vi "PTv3.0.vi"(8 "error in":errorcluster) -> ()   [LabVIEW 2017]
doc: "This VI runs in parallel to other tasks. It can contain as many user-defined periodic loops as you need. These can carry out PID or other sorts of timed response."
uses:
  <vilib>/Analysis/baseanly.llb/Mean (DBL).vi
  <vilib>/Rock Robotics/WPI/Utilities/WPI_GetSetVariantRefNum.vi
  <vilib>/Rock Robotics/Network Tables/NT Read Boolean.vi
  Robot Global Data.vi
  <vilib>/Rock Robotics/Network Tables/NT Write Number.vi
  <vilib>/Rock Robotics/Network Tables/NT Write Numeric Array.vi
  <vilib>/Analysis/NI_AALBase.lvlib
panel:
  out "Arrayval":dbl
  out "Accelerations":T1
  out "Joy Y":dbl(graph)
  out "Avg Y":dbl
  out "Mean":dbl(graph)
  out "Current Joy Y Value":dbl
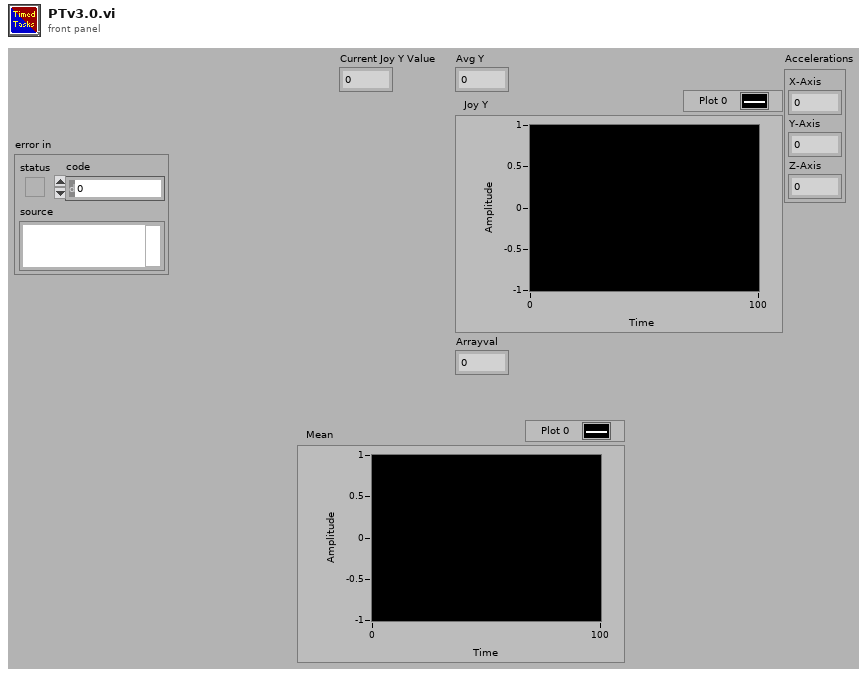
[diagram p1: front panel]
types:
  T1 = cluster{"X-Axis":dbl, "Y-Axis":dbl, "Z-Axis":dbl}
  T2 = typedef "WPI_JoystickDevRef.ctl" = cluster{"Device":T3}
  T3 = typedef "WPI_JoystickDeviceEnum.ctl" = enum16{"USB 0", "USB 1", "USB 2", "USB 3", "USB 4", "USB 5"}
  T4 = typedef "WPI_RobotDriveDevRef.ctl" = cluster{"DevStatus":errorcluster, "Motors[]":T5[], "Square Inputs":bool, "Max Output":dbl}
  T5 = typedef "WPI_MotorControlDeviceRef.ctl" = cluster{"DeviceStatus":errorcluster, "Type":T6, "PWM":cluster{"PWM Channel":T7, "DeadBand":T8}, "CAN":cluster{"Device Number":u8, "SetOutput VI Ref":variant, "GetOutput VI Ref":variant, "Enable VI Ref":variant, "Disable VI Ref":variant, "Data":variant}, "Invert":bool, "DIO PWM":cluster{"PWM \"Enable\" Channel":T7, "DIOChannel":T9, "PWM Rate":dbl}}
  T6 = typedef "WPI_MotorControlType.ctl" = enum16{"PWM", "CAN", "DIO PWM"}
  T7 = typedef "FPGA_DIOPWMChannel.ctl" = enum8{"PWM 0", "PWM 1", "PWM 2", "PWM 3", "PWM 4", "PWM 5", "PWM 6", "PWM 7", "PWM 8", "PWM 9", "PWM MXP 0", "PWM MXP 1", "PWM MXP 2", "PWM MXP 3", "PWM MXP 4", "PWM MXP 5", "PWM MXP 6", "PWM MXP 7", "PWM MXP 8", "PWM MXP 9", "Invalid"}
  T8 = typedef "WPI_PWMDeadband.ctl" = cluster{"Name":string, "maxPositivePwm":i32, "minPositivePwm":i32, "centerPwm":i32, "maxNegativePwm":i32, "minNegativePwm":i32, "angularRange":u16}
  T9 = typedef "FPGA_DIOChannel.ctl" = enum8{"DIO 0", "DIO 1", "DIO 2", "DIO 3", "DIO 4", "DIO 5", "DIO 6", "DIO 7", "DIO 8", "DIO 9", "DIO MXP 0", "DIO MXP 1", "DIO MXP 2", "DIO MXP 3", "DIO MXP 4", "DIO MXP 5", "DIO MXP 6", "DIO MXP 7", "DIO MXP 8", "DIO MXP 9", "DIO MXP 10", "DIO MXP 11", "DIO MXP 12", "DIO MXP 13", "DIO MXP 14", "DIO MXP 15", "SPI Port CS1", "SPI Port CS2", "SPI Port CS3", "SPI Port MISO", "SPI Port MOSI", "Invalid"}
  T10 = typedef "WPI_AccelerometerDevRef.ctl" = cluster{"DevStatus":errorcluster, "Scaling":T11, "Analog Channels":T12, "I2C Bus":T14, "SPI Bus":T15, "Accel Range":T16, "ADXL Axes":T17, "Handle":i32, "Device Address":u8, "Accel Type":enum16{"Analog", "ADXL345 I2C", "ADXL345 SPI", "Internal", "ADXL362 SPI"}}
  T11 = typedef "WPI_AccelerometerScaling.ctl" = cluster{"Gain (VoltsPerG)":dbl, "Center Voltage":dbl}
  T12 = typedef "WPI_AccelerometerAnalogChannels.ctl" = cluster{"X-Axis":T13, "Y-Axis":T13, "Z-Axis":T13}
  T13 = typedef "FPGA_AIChannel.ctl" = enum8{"AI 0", "AI 1", "AI 2", "AI 3", "AI MXP 0", "AI MXP 1", "AI MXP 2", "AI MXP 3", "Invalid"}
  T14 = typedef "i2c_bus.ctl" = enum16{"I2C On-Board", "I2C MXP", "Invalid"}
  T15 = typedef "spi_bus.ctl" = enum16{"SPI On-Board, CS0", "SPI On-Board, CS1", "SPI On-Board, CS2", "SPI On-Board, CS3", "SPI MXP", "Invalid"}
  T16 = typedef "ADXL345 Range.ctl" = u8
  T17 = typedef "WPI_AccelerometerADXL345 Axes.ctl" = cluster{"X-Axis":bool, "Y-Axis":bool, "Z-Axis":bool}
  T18 = typedef "WPI_GyroDevRef.ctl" = cluster{"DevStatus":errorcluster, "Analog Channel":T13, "Gain (VoltsPerDegree/Second)":dbl, "Gyro Type":enum16{"Analog", "XRS450"}, "Handle":i32, "SPI Bus":T15, "Device Found":bool, "Sample Rate":dbl, "Calibrate On Open":bool, "Offset":dbl}
  T19 = cluster{"JoystickDevRef":T2, "RobotDriveDevRef":T4}
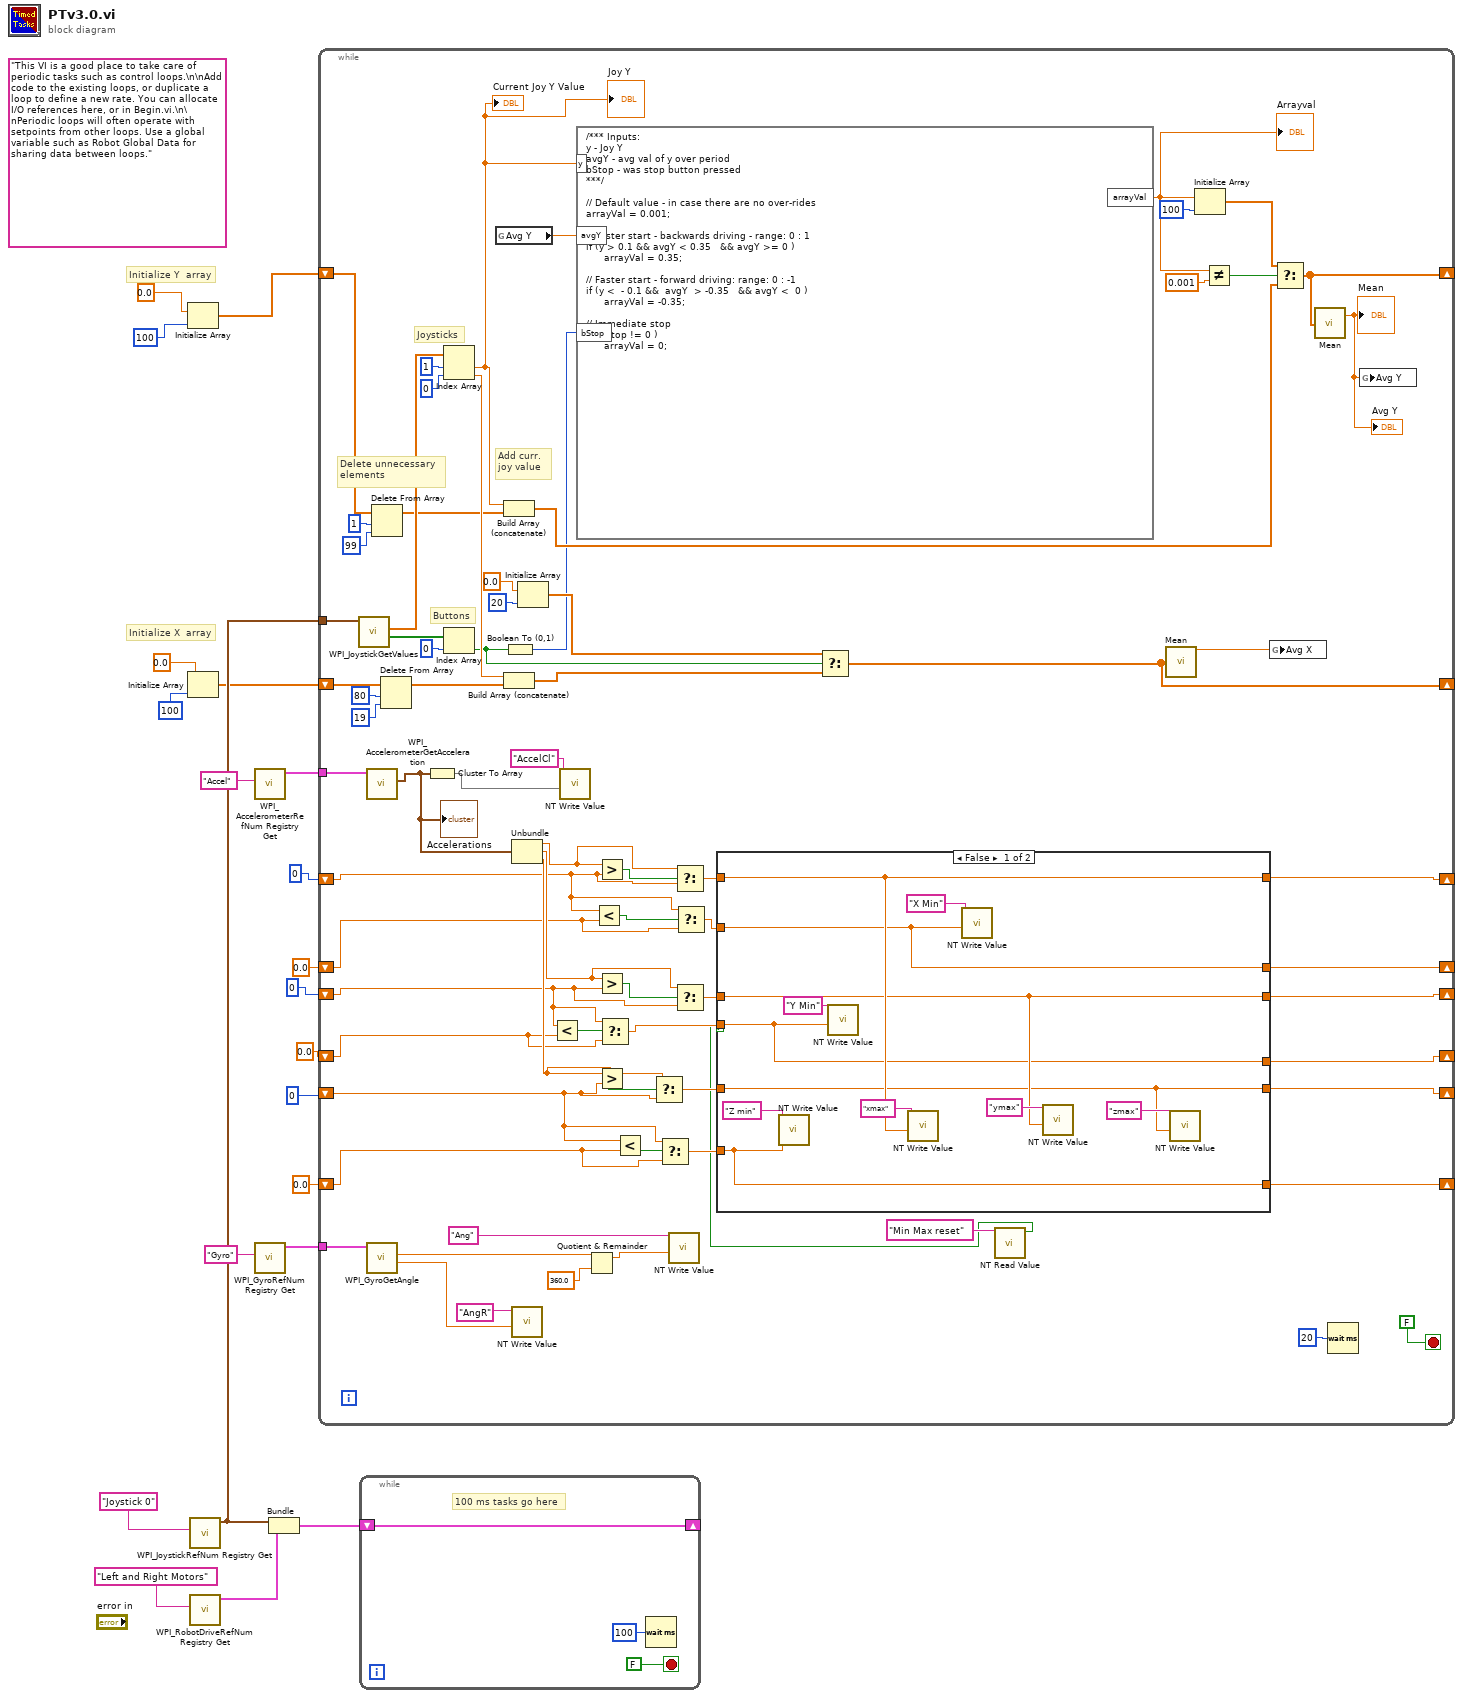
[diagram p0: block diagram]
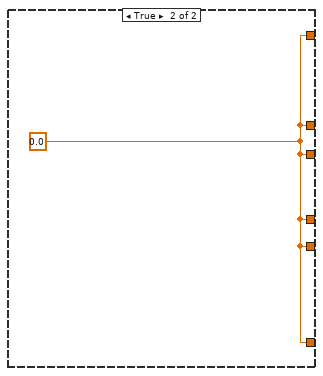
[diagram p2: hidden frame]
diagram:
  (unwired) "This VI is a good place to take care of periodic tasks such as control loops.\n\nAdd code to the existing loops, or duplicate a loop to define a new rate. You can allocate I/O references here, or in Begin.vi.\n\nPeriodic loops will often operate with setpoints from other loops. Use a global variable such as Robot Global Data for sharing data between loops."
  # "Initialize X  array"
  # "Initialize Y  array"
  n1 = Initialize Array(0.0 ("element"), 100 ("dimension size")) -> (w14:dbl[])
  n2 = Initialize Array(0.0 ("element"), 100 ("dimension size")) -> (w13:dbl[])
  n3 = call <vilib>:"WPI_JoystickRefNum Registry Get.vi"("refnum name"="Joystick 0") -> ("JoystickDevRef"=w17:T2)  [unwired: 1 in, 9 out]
  n4 = call <vilib>:"WPI_RobotDriveRefNum Registry Get.vi"("refnum name"="Left and Right Motors") -> ("RobotDriveDevRef"=w19:T4)  [unwired: 1 in, 9 out]
  n5 = call <vilib>:"WPI_AccelerometerRefNum Registry Get.vi"("refnum name"="Accel") -> ("AccelerometerDevRef"=w9:T10)  [unwired: 9 in, 1 out]
  n6 = call <vilib>:"WPI_GyroRefNum Registry Get.vi"("refnum name"="Gyro") -> ("GyroDevRef"=w7:T18)  [unwired: 9 in, 1 out]
  n7 = Bundle("JoystickDevRef"=w17, "RobotDriveDevRef"=w19) -> (w18:T19)  [unwired: 1 out]
  n8 = while {
    tunnel: w17 -> [w94]
    shift-right: [w68] -> _
    shift-left: w14 -> [w91]
    shift-right: [w87] -> _
    shift-left: w13 -> [w81]
    tunnel: w9 -> [w63]
    tunnel: w7 -> [w62]
    shift-right: [w28] -> _
    shift-left: 0 -> [w41]
    shift-right: [w26] -> _
    shift-left: 0 -> [w37]
    shift-right: [w24] -> _
    shift-left: 0 -> [w34]
    shift-right: [w27] -> _
    shift-left: 0.0 ("X-Axis") -> [w39]
    shift-right: [w25] -> _
    shift-left: 0.0 ("Y-Axis") -> [w35]
    shift-right: [w23] -> _
    shift-left: 0.0 ("Z-Axis") -> [w31]
    stop <- FALSE stop-if-true
    # "Add curr. \njoy value"
    # "Delete unnecessary \nelements"
    # "Joysticks"
    # "Buttons"
    n9 = call <vilib>:"WPI_JoystickGetValues.vi"("JoystickDevRef"=w94) -> ("Buttons"=w90:bool[], "Axes"=w93:dbl[])  [unwired: 6 in, 3 out]
    n10 = call <vilib>:"WPI_AccelerometerGetAcceleration.vi"("AccelerometerDevRef"=w63) -> ("Accelerations"=w53:T1)  [unwired: 8 in, 2 out]
    "Accelerations" <- w53
    n11 = call <vilib>:"WPI_GyroGetAngle.vi"("GyroDevRef"=w62) -> ("Angular Rate"=w60:dbl, "Angle"=w55:dbl)  [unwired: 6 in, 3 out]
    n12 = Delete From Array(array=w91, length=1, index=99) -> (array with subset deleted=w73:dbl[])  [unwired: 1 out]
    n13 = Delete From Array(array=w81, length=80, index=19) -> (array with subset deleted=w83:dbl[])  [unwired: 1 out]
    n14 = Cluster To Array(cluster=w53) -> (array=w61:dbl[])
    n15 = Index Array(array=w93, index #1=1 ("index"), index #2=0 ("index")) -> (element #1=w64:dbl, element #2=w79:dbl)
    "Current Joy Y Value" <- w64
    "Joy Y" <- w64
    n16 = Index Array(array=w90, index=0) -> (element=w69:bool)
    n17 = global read "Robot Global Data.vi" "Avg Y"() -> (w71:dbl)
    n18 = Build Array (concatenate)(w64, w73) -> (w72:dbl[])
    n19 = Build Array (concatenate)(w79, w83) -> (w80:dbl[])
    n20 = Boolean To (0,1)(Boolean=w69) -> (0, 1=w70:i16)
    n21 = Unbundle(w53) -> ("X-Axis"=w51:dbl, "Y-Axis"=w48:dbl, "Z-Axis"=w47:dbl)
    n22 = call-poly <vilib>:"NT Write Value.vi"("Numeric"=w60, "Name"="AngR") -> ()  [unwired: 9 in, 1 out]
    n23 = Initialize Array(0.0 ("element"), 20 ("dimension size")) -> (w86:dbl[])
    n24 = Less?(x=w37, y=w35) -> (x < y?=w38:bool)
    n25 = call-poly <vilib>:"NT Write Value.vi"("Numeric Array"=w61, "Name"="AccelCl") -> ()  [unwired: 9 in, 1 out]
    n26 = formula code="/*** Inputs:\ny - Joy Y\navgY - avg val of y over period\nbStop - was stop button pressed\n***/\n\n// Default value - in case there are no over-rides\narrayVal = 0.001;\n\n// Faster start - backwards driving - range: 0 : 1\nif (y > 0.1 && avgY < 0.35   && avgY >= 0 )\n      arrayVal = 0.35;\n\n// Faster start - forward driving: range: 0 : -1\nif (y <  - 0.1 &&  avgY  > -0.35   && avgY <  0 )\n      arrayVal = -0.35;\n\n// Immediate stop\nif (bStop != 0 )\n      arrayVal = 0;"("y"=w64, "avgY"=w71, "bStop"=w70) -> ("arrayVal"=w65:dbl)
    "Arrayval" <- w65
    n27 = Quotient & Remainder(x=w55, y=360.0) -> (x-y*floor(x/y)=w54:dbl)  [unwired: 1 out]
    n28 = Less?(x=w41, y=w39) -> (x < y?=w42:bool)
    n29 = Greater?(x=w51, y=w41) -> (0:w52:bool)
    n30 = Greater?(x=w48, y=w37) -> (0:w50:bool)
    n31 = Greater?(x=w47, y=w34) -> (0:w49:bool)
    n32 = Select(t=w37, s=w38, f=w35) -> (s? t:f=w36:dbl)
    n33 = Less?(x=w34, y=w31) -> (x < y?=w33:bool)
    n34 = Select(t=w47, s=w49, f=w34) -> (s? t:f=w45:dbl)
    n35 = Select(t=w34, s=w33, f=w31) -> (s? t:f=w32:dbl)
    n36 = call-poly <vilib>:"NT Write Value.vi"("Numeric"=w54, "Name"="Ang") -> ()  [unwired: 9 in, 1 out]
    n37 = Select(t=w51, s=w52, f=w41) -> (s? t:f=w46:dbl)
    n38 = Select(t=w48, s=w50, f=w37) -> (s? t:f=w29:dbl)
    n39 = Select(t=w41, s=w42, f=w39) -> (s? t:f=w40:dbl)
    n40 = Select(t=w86, s=w69, f=w80) -> (s? t:f=w87:dbl[])
    n41 = call-poly <vilib>:"NT Read Value.vi"("Name"="Min Max reset") -> ("Boolean"=w22:bool)  [unwired: 9 in, 1 out]
    n42 = case shown="False" w22 {
      tunnel: w46 -> [w102 _]
      tunnel: w29 -> [w100 _]
      tunnel: w45 -> [w98 _]
      tunnel: w40 -> [w101 _]
      tunnel: w36 -> [w99 _]
      tunnel: w32 -> [w97 _]
      tunnel: [w102 w109] -> w28
      tunnel: [w101 w109] -> w27
      tunnel: [w100 w109] -> w26
      tunnel: [w99 w109] -> w25
      tunnel: [w98 w109] -> w24
      tunnel: [w97 w109] -> w23
      frame False {
        n43 = call-poly <vilib>:"NT Write Value.vi"("Numeric"=w97, "Name"="Z min") -> ()  [unwired: 9 in, 1 out]
        n44 = call-poly <vilib>:"NT Write Value.vi"("Numeric"=w99, "Name"="Y Min") -> ()  [unwired: 9 in, 1 out]
        n45 = call-poly <vilib>:"NT Write Value.vi"("Numeric"=w102, "Name"="xmax") -> ()  [unwired: 9 in, 1 out]
        n46 = call-poly <vilib>:"NT Write Value.vi"("Numeric"=w101, "Name"="X Min") -> ()  [unwired: 9 in, 1 out]
        n47 = call-poly <vilib>:"NT Write Value.vi"("Numeric"=w100, "Name"="ymax") -> ()  [unwired: 9 in, 1 out]
        n48 = call-poly <vilib>:"NT Write Value.vi"("Numeric"=w98, "Name"="zmax") -> ()  [unwired: 9 in, 1 out]
      }
      frame True {
        w109 = 0.0
      }
    }
    n49 = call-poly <vilib>:"Mean.vi"("X"=w87) -> ("mean"=w44:dbl)  [unwired: 1 out]
    n50 = Initialize Array(w65, 100 ("dimension size")) -> (w75:dbl[])
    n51 = Not Equal?(x=w65, y=0.001) -> (x != y?=w67:bool)
    n52 = global write "Robot Global Data.vi" "Avg X"(w44) -> ()
    n53 = Select(t=w75, s=w67, f=w72) -> (s? t:f=w68:dbl[])
    n54 = call-poly <vilib>:"Mean.vi"("X"=w68) -> ("mean"=w43:dbl)  [unwired: 1 out]
    "Mean" <- w43
    "Avg Y" <- w43
    n55 = Wait (ms)(milliseconds to wait=u32 20) -> ()  [unwired: 1 out]
    n56 = global write "Robot Global Data.vi" "Avg Y"(w43) -> ()
  }
  n57 = while {
    shift-right: [w110] -> _
    shift-left: w18 -> [w110]
    stop <- FALSE stop-if-true
    # "100 ms tasks go here"
    n58 = Wait (ms)(milliseconds to wait=u32 100) -> ()  [unwired: 1 out]
  }
